vi "S7COMM - Evaluate Response Item Return Code.vi"(8 "error in (no error)":errorcluster, 11 "Return Code":T1 format="0x%02x") -> (0 "error out":errorcluster)   [LabVIEW 2014, in "S7NetCom.lvclass"]
uses:
  S7NetCom.lvclass
  Controls/S7NetCom_HexByte.ctl
  S7COMM - Response Item Return Codes--ring.ctl
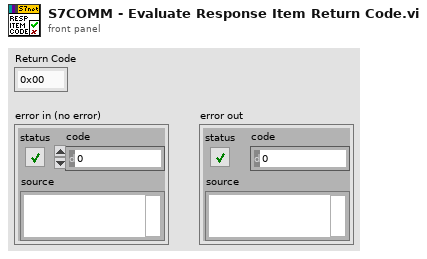
[diagram p1: front panel]
types:
  T1 = typedef "S7NetCom.lvclass/S7NetCom_HexByte.ctl" = u8
  T2 = typedef "S7NetCom.lvclass/S7COMM - Response Item Return Codes--ring.ctl" = enum16{"Reserved (0x00)", "Hardware Fault (0x01)", "Object Access Violation (0x03)", "Address Out of Range (0x05)", "Unsupported Data Type (0x06)", "Inconsistent Data Type (size mismatch?) (0x07)", "Object does not exist (0x0A)", "Success (0xFF)"}
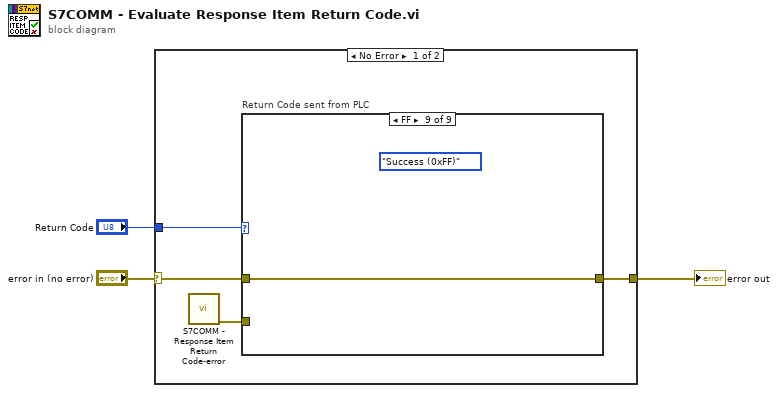
[diagram p0: block diagram]
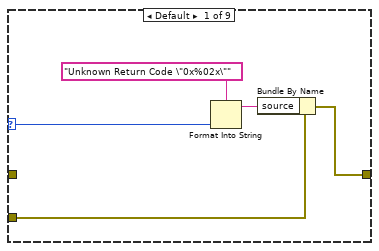
[diagram p2: hidden frame]
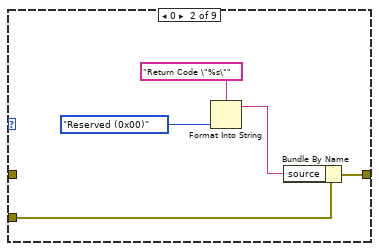
[diagram p3: hidden frame]
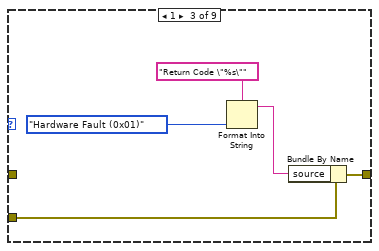
[diagram p4: hidden frame]
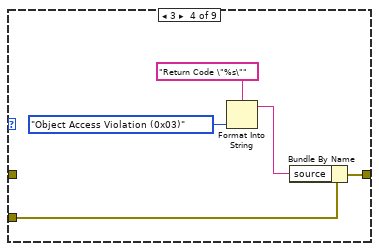
[diagram p5: hidden frame]
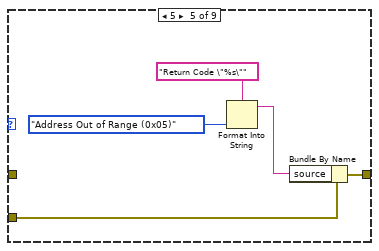
[diagram p6: hidden frame]
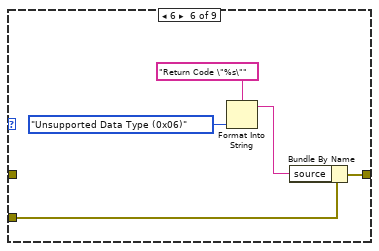
[diagram p7: hidden frame]
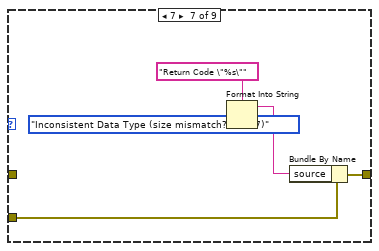
[diagram p8: hidden frame]
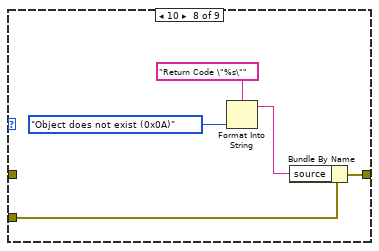
[diagram p9: hidden frame]
diagram:
  n1 = case shown="No Error" "error in (no error)" {
    selector: "error in (no error)" -> [w6 w49]
    tunnel: [w5 w49] -> w3
    tunnel: "Return Code" -> [w7 _]
    frame No Error {
      n2 = call "S7COMM - Response Item Return Code-error.vi"() -> ("error out"=w4:errorcluster)  [unwired: 11 in]
      n3 = case "Return Code sent from PLC" shown="FF" w7 {
        selector: w7 -> [w8 _ _ _ _ _ _ _ _]
        tunnel: w6 -> [_ _ _ _ _ _ _ _ w48]
        tunnel: [w11 w16 w21 w26 w31 w36 w41 w46 w48] -> w5
        tunnel: w4 -> [w12 w17 w22 w27 w32 w37 w42 w47 _]
        frame Default {
          n4 = Format Into String(format string="Unknown Return Code \"0x%02x\"", w8) -> (resulting string=w10:string)  [unwired: 2 in, 1 out]
          n5 = Bundle By Name(cluster=w12, "source"=w10) -> (w11:errorcluster)
        }
        frame 0 {
          n6 = Format Into String(format string="Return Code \"%s\"", S7COMM_-_Response_Item_Return_Codes--ring."Reserved (0x00)" ("Response Item Return Codes")) -> (resulting string=w15:string)  [unwired: 2 in, 1 out]
          n7 = Bundle By Name(cluster=w17, "source"=w15) -> (w16:errorcluster)
        }
        frame 1 {
          n8 = Format Into String(format string="Return Code \"%s\"", S7COMM_-_Response_Item_Return_Codes--ring."Hardware Fault (0x01)" ("Response Item Return Codes")) -> (resulting string=w20:string)  [unwired: 2 in, 1 out]
          n9 = Bundle By Name(cluster=w22, "source"=w20) -> (w21:errorcluster)
        }
        frame 3 {
          n10 = Format Into String(format string="Return Code \"%s\"", S7COMM_-_Response_Item_Return_Codes--ring."Object Access Violation (0x03)" ("Response Item Return Codes")) -> (resulting string=w25:string)  [unwired: 2 in, 1 out]
          n11 = Bundle By Name(cluster=w27, "source"=w25) -> (w26:errorcluster)
        }
        frame 5 {
          n12 = Format Into String(format string="Return Code \"%s\"", S7COMM_-_Response_Item_Return_Codes--ring."Address Out of Range (0x05)" ("Response Item Return Codes")) -> (resulting string=w30:string)  [unwired: 2 in, 1 out]
          n13 = Bundle By Name(cluster=w32, "source"=w30) -> (w31:errorcluster)
        }
        frame 6 {
          n14 = Format Into String(format string="Return Code \"%s\"", S7COMM_-_Response_Item_Return_Codes--ring."Unsupported Data Type (0x06)" ("Response Item Return Codes")) -> (resulting string=w35:string)  [unwired: 2 in, 1 out]
          n15 = Bundle By Name(cluster=w37, "source"=w35) -> (w36:errorcluster)
        }
        frame 7 {
          n16 = Format Into String(format string="Return Code \"%s\"", S7COMM_-_Response_Item_Return_Codes--ring."Inconsistent Data Type (size mismatch?) (0x07)" ("Response Item Return Codes")) -> (resulting string=w40:string)  [unwired: 2 in, 1 out]
          n17 = Bundle By Name(cluster=w42, "source"=w40) -> (w41:errorcluster)
        }
        frame 10 {
          n18 = Format Into String(format string="Return Code \"%s\"", S7COMM_-_Response_Item_Return_Codes--ring."Object does not exist (0x0A)" ("Response Item Return Codes")) -> (resulting string=w45:string)  [unwired: 2 in, 1 out]
          n19 = Bundle By Name(cluster=w47, "source"=w45) -> (w46:errorcluster)
        }
        frame 255 {
          (unwired) S7COMM_-_Response_Item_Return_Codes--ring."Success (0xFF)" ("Response Item Return Codes")
        }
      }
    }
    frame Error {
    }
  }
  "error out" <- w3
